vi "command_get_current_position.vi"(8 "error in (no error)":errorcluster, 11 "StageMH110930Scientifica in":refnum<class "StageMH110930Scientifica.lvclass">) -> (0 "error out":errorcluster, 2 "current position":refnum<class "SpaceVector.lvclass">, 3 "StageMH110930Scientifica out":refnum<class "StageMH110930Scientifica.lvclass">)   [LabVIEW 2010, in "StageMH110930Scientifica.lvclass"]
uses:
  StageMH110930Scientifica.lvclass
  common/classes/SpaceVector/SpaceVector/SpaceVector.lvclass
  common/classes/ErrorController/ErrorController/class_data.vi
  common/classes/ErrorController/ErrorController/ErrorController.lvclass
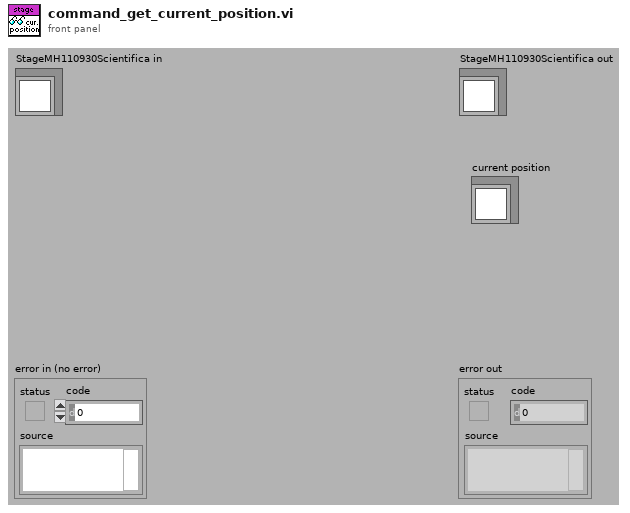
[diagram p1: front panel]
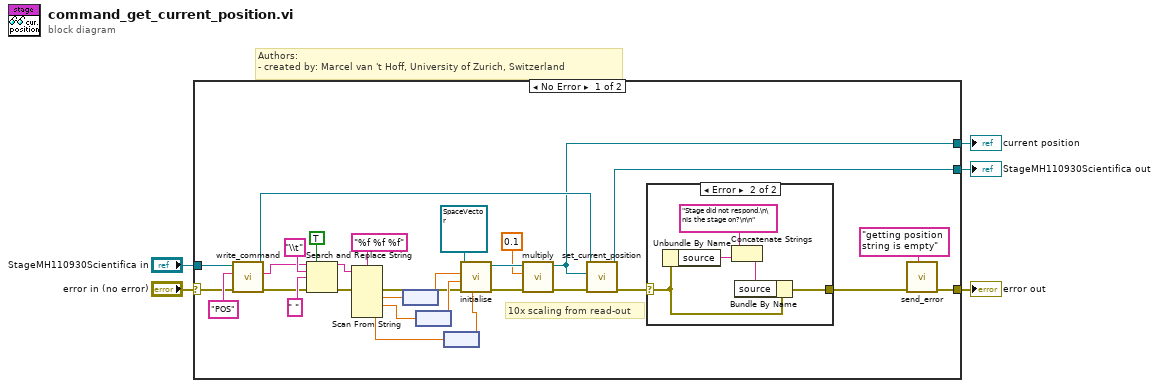
[diagram p0: block diagram]
diagram:
  # "Authors: \n- created by: Marcel van 't Hoff, University of Zurich, Switzerland"
  n1 = case shown="No Error" "error in (no error)" {
    selector: "error in (no error)" -> [w31 w43]
    tunnel: [w9 w43] -> w4
    tunnel: [w32 w42] -> w2
    tunnel: "StageMH110930Scientifica in" -> [w35 w42]
    tunnel: [w13 _] -> w1
    frame No Error {
      # "10x scaling from read-out"
      n2 = call-dynamic "write_command.vi"("error in (no error)"=w31, "string to write"="POS", "StageMH110930Scientifica in"=w35) -> ("error out"=w17:errorcluster, "read string"=w16:string, "StageMH110930Scientifica out"=w33:refnum<class "StageMH110930Scientifica.lvclass">)  [unwired: 5 in, 1 out]
      n3 = Search and Replace String(replace all?=TRUE ("replace all? (F)"), input string=w16, search string="\\t", replace string=" " ("replace string (\"\")"), error in=w17) -> (result string=w19:string, error out=w15:errorcluster)  [unwired: 3 in, 2 out]
      n4 = Scan From String(format string="%f %f %f", input string=w19, error in=w15) -> (error out=w22:errorcluster, output 1=w29:dbl, output 2=w28:dbl, output 3=w27:dbl)  [unwired: 1 in, 5 out]
      n5 = node(w29) -> (w26:dbl[unit])
      n6 = node(w28) -> (w25:dbl[unit])
      n7 = node(w27) -> (w24:dbl[unit])
      n8 = call "initialise.vi"("z"=w24, "error in (no error)"=w22, "y"=w25, "x"=w26, "SpaceVector in"=refnum<class "SpaceVector.lvclass"> refnum) -> ("error out"=w12:errorcluster, "SpaceVector out"=w14:refnum<class "SpaceVector.lvclass">)  [unwired: 5 out]
      n9 = call "multiply.vi"("error in (no error)"=w12, "factor"=0.1, "SpaceVector in"=w14) -> ("error out"=w11:errorcluster, "SpaceVector out"=w13:refnum<class "SpaceVector.lvclass">)  [unwired: 7 in]
      n10 = call-dynamic "set_current_position.vi"("error in (no error)"=w11, "current position"=w13, "DL090409StageScaffold.lvclass in"=w33) -> ("error out"=w7:errorcluster, "DL090409StageScaffold.lvclass out"=w32:refnum<class "StageMH110930Scientifica.lvclass">)  [unwired: 7 out]
      n11 = case shown="Error" w7 {
        selector: w7 -> [w36 w41]
        tunnel: [w36 w40] -> w6
        frame No Error {
        }
        frame Error {
          n12 = Unbundle By Name(w41) -> ("source"=w38:string)
          n13 = Concatenate Strings("Stage did not respond.\n\nIs the stage on?\n\n" ("string"), w38) -> (w39:string)
          n14 = Bundle By Name(cluster=w41, "source"=w39) -> (w40:errorcluster)
        }
      }
      n15 = call "send_error.vi"("additional message"="getting position string is empty", "error in (no error)"=w6) -> ("error out"=w9:errorcluster)  [unwired: 9 in]
    }
    frame Error {
    }
  }
  "error out" <- w4
  "StageMH110930Scientifica out" <- w2
  "current position" <- w1
